vi "Gyro.vi"() -> (0 "Dis":bool, 1 "Dir":bool)   [LabVIEW 2016]
uses:
  <vilib>/Rock Robotics/Network Tables/NT Read Boolean.vi
  <vilib>/Rock Robotics/Network Tables/NT Read Number.vi
  <vilib>/Rock Robotics/WPI/ThirdParty/Sensors/ADIS16448 IMU/ADIS16448_IMU.lvlib
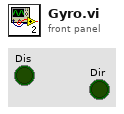
[diagram p1: front panel]
types:
  T1 = typedef "ADIS16448_IMU.lvlib/ADI_IMU_ADIS16448_InterruptDevRef.ctl" = cluster{"ADI IMU DevRef":T2, "InterruptRef":T4}
  T2 = typedef "ADIS16448_IMU.lvlib/ADI_IMU_ADIS16448_IMUDevRef.ctl" = cluster{"DevStatus":errorcluster, "Handle":i32, "SPI Bus":T3, "Device Found":bool, "Device Ready":bool, "Yaw Axis":enum16{"X", "Y", "Z"}, "AHRS Algorithm":enum16{"Complementary", "Madgwick"}, "Serial":u16, "Lot ID 2":u16, "Lot ID 1":u16, "Product ID":u16}
  T3 = typedef "spi_bus.ctl" = enum16{"SPI On-Board, CS0", "SPI On-Board, CS1", "SPI On-Board, CS2", "SPI On-Board, CS3", "SPI MXP", "Invalid"}
  T4 = typedef "WPI_InterruptRef.ctl" = cluster{"DevStatus":errorcluster, "InterruptIndex":T5}
  T5 = typedef "FPGA_InterruptIndex.ctl" = enum8{"0", "1", "2", "3", "4", "5", "6", "7", "Invalid"}
  T6 = cluster{"X Angle":dbl, "Y Angle":dbl, "Z Angle":dbl}
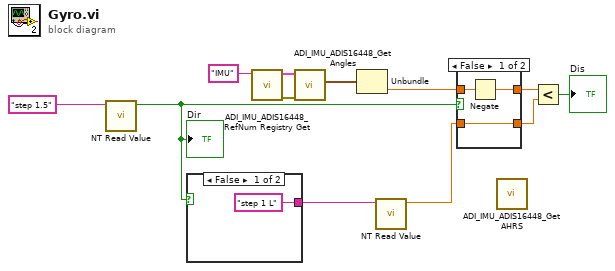
[diagram p0: block diagram]
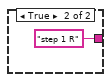
[diagram p2: hidden frame]
diagram:
  n1 = call-poly <vilib>:"NT Read Value.vi"("Name"="step 1.5") -> ("Boolean"=w1:bool)  [unwired: 9 in, 1 out]
  "Dir" <- w1
  n2 = case shown="False" w1 {
    tunnel: ["step 1 L" ("Name") "step 1 R" ("Name")] -> w12
    frame False {
    }
    frame True {
    }
  }
  n3 = call <vilib>:"ADI_IMU_ADIS16448_RefNum Registry Get.vi"("refnum name"="IMU") -> ("error out"=w7:errorcluster, "ADI IMU Interrupt DevRef"=w8:T1)  [unwired: 9 in]
  n4 = call <vilib>:"ADI_IMU_ADIS16448_Get Angles.vi"("error in"=w7, "ADI IMU Interrupt DevRef"=w8) -> ("IMU Angles Out"=w6:T6)  [unwired: 6 in, 3 out]
  n5 = Unbundle(w6) -> ("Z Angle"=w5:dbl)  [unwired: 2 out]
  n6 = call-poly <vilib>:"NT Read Value.vi"("Name"=w12) -> ("Numeric"=w10:dbl)  [unwired: 9 in, 1 out]
  n7 = case shown="False" w1 {
    tunnel: w5 -> [w17 w19]
    tunnel: [w16 w19] -> w11
    tunnel: w10 -> [w15 w18]
    tunnel: [w15 w18] -> w9
    frame False {
      n8 = Negate(x=w17) -> (-x=w16:dbl)
    }
    frame True {
    }
  }
  n9 = call <vilib>:"ADI_IMU_ADIS16448_Get AHRS.vi"() -> ()  [unwired: 7 in, 5 out]
  n10 = Less?(x=w11, y=w9) -> (x < y?=→"Dis":bool)
